vi "miniUSB_pulseCheck_query_ACF.vi"() -> ()   [LabVIEW 2013]
uses:
  tcp client action.ctl
panel:
  out "ACF":cluster{dbl[], dbl[]}(graph)
  out "FWHM":dbl
  out "Device Info":string
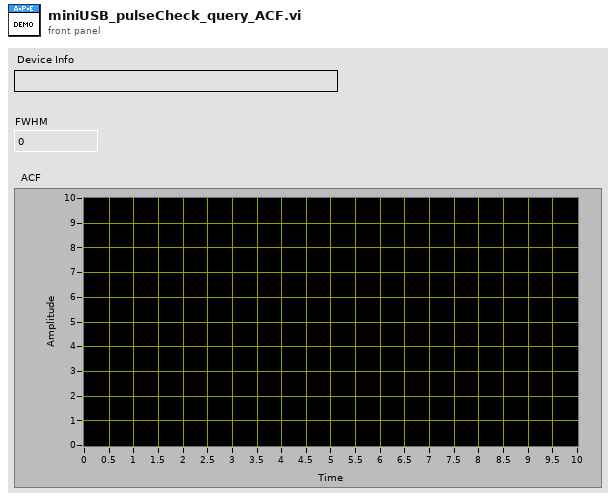
[diagram p1: front panel]
types:
  T1 = typedef "tcp client action.ctl" = enum16{"Connect", "Write", "Query", "Disconnect"}
  T2 = enum16{"big-endian, network order", "native, host order", "little-endian"}
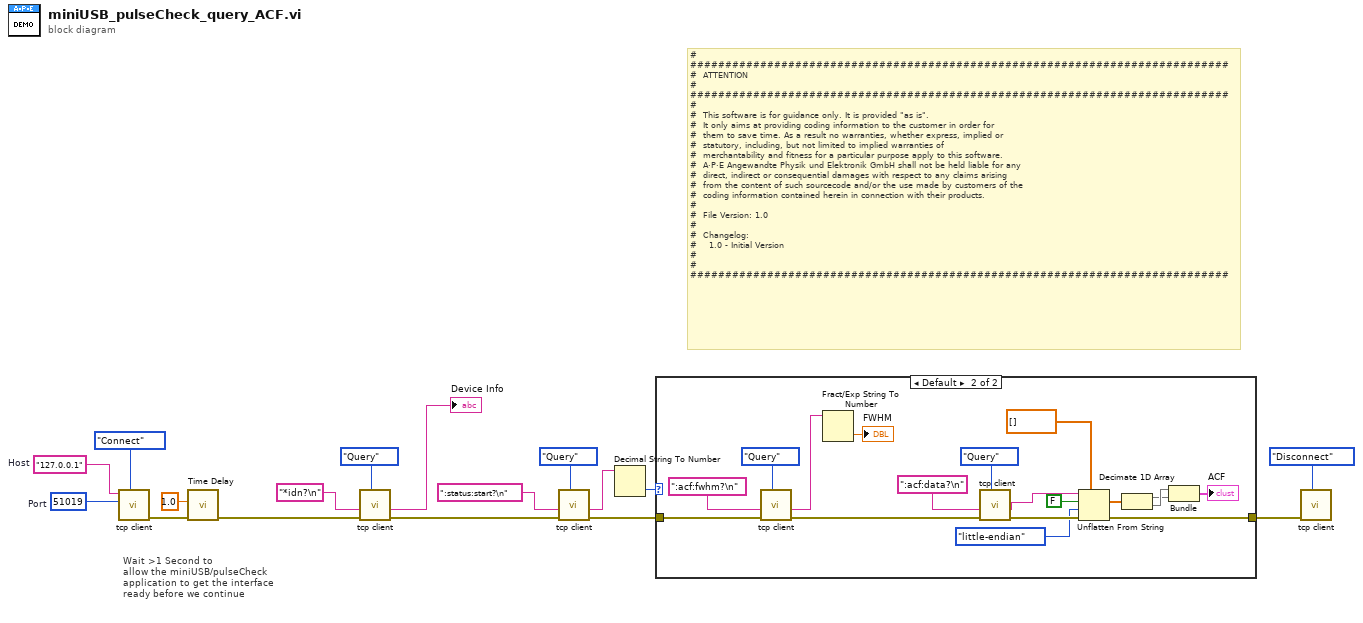
[diagram p0: block diagram]
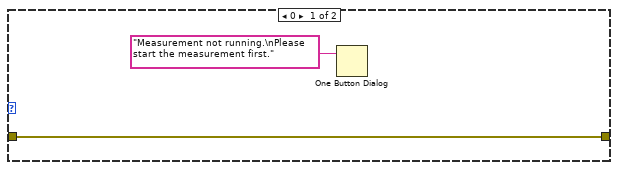
[diagram p2: hidden frame]
diagram:
  w16 = u16 51019  # Port
  w15 = "127.0.0.1"  # Host
  # "Wait >1 Second to\nallow the miniUSB/pulseCheck\napplication to get the interface\nready before we continue"
  # "# #############################################################################\n#  ATTENTION\n# #############################################################################\n#\n#  This software is for guidance only. It is provided \"as is\".\n#  It only aims at providing coding information to the customer in order for\n#  them to save time. As a result no warranties, whether express, implied or\n#  statutory, including, but not limited to implied warranties of\n#  merchantability and fitness for a particular purpose apply to this software.\n#  A·P·E Angewandte Physik und Elektronik GmbH shall not be held liable for any\n#  direct, indirect or consequential damages with respect to any claims arising\n#  from the content of such sourcecode and/or the use made by customers of the\n#  coding information contained herein in connection with their products.\n#\n#  File Version: 1.0\n#\n#  Changelog:\n#    1.0 - Initial Version\n#\n# #############################################################################"
  n1 = call "tcp client.vi"("Action"=tcp_client_action."Connect", "TCP Port"=w16, "Host"=w15) -> ("error out"=w3:errorcluster)  [unwired: 7 in, 1 out]
  n2 = call "Time Delay"("error in (no error)"=w3, "Delay Time (s)"=1.0) -> ("error out"=w2:errorcluster)  [unwired: 9 in]
  n3 = call "tcp client.vi"("Action"=tcp_client_action."Query", "error in"=w2, "Command"="*idn?\n") -> ("error out"=w9:errorcluster, "Answer"=→"Device Info":string)  [unwired: 7 in]
  n4 = call "tcp client.vi"("Action"=tcp_client_action."Query", "error in"=w9, "Command"=":status:start?\n") -> ("error out"=w7:errorcluster, "Answer"=w8:string)  [unwired: 7 in]
  n5 = Decimal String To Number(string=w8) -> (number=w6:i32)  [unwired: 2 in, 1 out]
  n6 = case shown="Default" w6 {
    tunnel: w7 -> [w18 w35]
    tunnel: [w18 w24] -> w4
    frame 0 {
      n7 = One Button Dialog(message="Measurement not running.\nPlease start the measurement first.") -> ()  [unwired: 1 in, 1 out]
    }
    frame Default {
      n8 = call "tcp client.vi"("Action"=tcp_client_action."Query", "error in"=w35, "Command"=":acf:fwhm?\n") -> ("error out"=w30:errorcluster, "Answer"=w37:string)  [unwired: 7 in]
      n9 = Fract/Exp String To Number(string=w37) -> (number=→"FWHM":dbl)  [unwired: 3 in, 1 out]
      n10 = call "tcp client.vi"("Action"=tcp_client_action."Query", "error in"=w30, "Command"=":acf:data?\n") -> ("error out"=w29:errorcluster, "Answer"=w28:string)  [unwired: 7 in]
      n11 = Unflatten From String(type=dbl[] [], binary string=w28, data includes array or string size? (T)=FALSE, byte order (0:big-endian, network order)=T2."little-endian", error in (no error)=w29) -> (value=w23:dbl[], error out=w24:errorcluster)  [unwired: 1 out]
      n12 = Decimate 1D Array(w23) -> (w20:dbl[], w21:dbl[])
      n13 = Bundle(w21, w20) -> (→"ACF":cluster{dbl[], dbl[]})  [unwired: 1 in]
    }
  }
  n14 = call "tcp client.vi"("Action"=tcp_client_action."Disconnect", "error in"=w4) -> ()  [unwired: 8 in, 2 out]
